vi "Inventario--constant.vi"() -> (3 "Path":path)   [LabVIEW 2024, in "ProductControl.lvlib"]
uses:
  ProductControl.lvlib
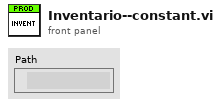
[diagram p1: front panel]
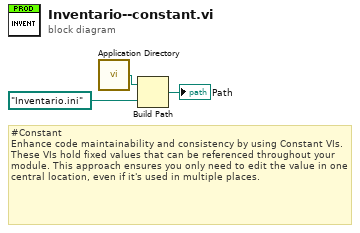
[diagram p0: block diagram]
diagram:
  # "#Constant\nEnhance code maintainability and consistency by using Constant VIs. These VIs hold fixed values that can be referenced throughout your module. This approach ensures you only need to edit the value in one central location, even if it's used in multiple places."
  n1 = call <vilib>:"Application Directory.vi"() -> ("Application Directory"=w3:path)
  n2 = Build Path(base path=w3, name or relative path=path "Inventario.ini") -> (appended path=→"Path":path)
